vi "DG535.get D Delay.vi"(0 "i ref in":refnum<vi>, 11 "error in (no error)":errorcluster) -> (4 "i ref out":refnum<vi>, 6 "D=":i32(slide) scale=0.0..3.0, 8 "D":dbl min=0.0 max=999.999999999995 format="%.12f", 10 "Ref Channel":string, 15 "error out":errorcluster)   [LabVIEW 2014, in "DG535.lvlib"]
uses:
  DG535.lvlib
panel:
  # "+"
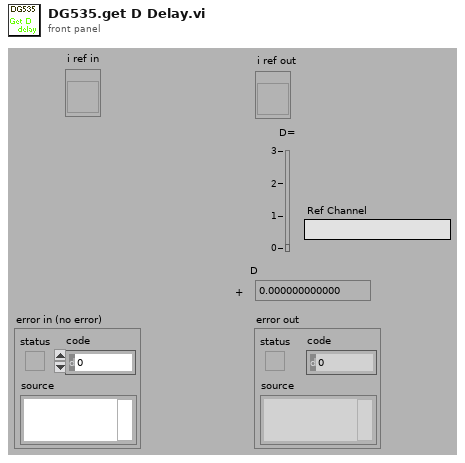
[diagram p1: front panel]
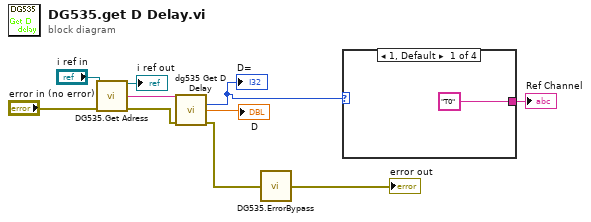
[diagram p0: block diagram]
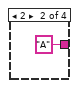
[diagram p2: hidden frame]
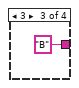
[diagram p3: hidden frame]
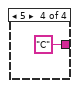
[diagram p4: hidden frame]
diagram:
  n1 = call "DG535.Get Adress.vi"("i ref in"="i ref in", "error in (no error)"="error in (no error)") -> ("i ref out"=→"i ref out":refnum<vi>, "address"=w6:string, "error out"=w5:errorcluster)  [unwired: 10 in, 1 out]
  n2 = call "dg535 Get D Delay.vi"("address string"=w6, "error in"=w5) -> ("D="=w3:i32, "D"=→"D":dbl, "error out"=w4:errorcluster)  [unwired: 11 in]
  "D=" <- w3
  n3 = call "DG535.ErrorBypass.vi"("error in (no error)"=w4) -> ("error out"=→"error out":errorcluster)  [unwired: 14 in]
  n4 = case shown="1, Default" w3 {
    tunnel: ["T0" "A" "B" "C"] -> w2
    frame 1, Default {
    }
    frame 2 {
    }
    frame 3 {
    }
    frame 5 {
    }
  }
  "Ref Channel" <- w2
